vi "edit.vi"(8 "error in (no error)":errorcluster, 11 "TCSettings in":refnum<class "TCSettings.lvclass">) -> (0 "error out":errorcluster, 2 "cancelIsTrue out":bool, 3 "TCSettings out":refnum<class "TCSettings.lvclass">)   [LabVIEW 2016, in "Settings.lvlib" / "TCSettings.lvclass"]
uses:
  TCSettings.lvclass
  C:/Users/aanania/Documents/ts_monochromator_windows/MonoSettings/Settings/Settings/Setting.lvclass
  ConfigurationTypedefs/Base/MonochromatorSettings.ctl
  Typedefs/wavelength.ctl
  Typedefs/slitWidth.ctl
  ConfigurationTypedefs/Base/TCPConfiguration.ctl
  Settings/Setting.lvclass/Setting.ctl
  <vilib>/Utility/xml.llb/Write to XML File(string).vi
  Settings/Setting.lvclass
  ConfigurationTypedefs/ConfigurationTypedefs.lvlib
panel:
  in  "SettingTab":enum32{"TCP Settings", "Monochromator Limits"}(tab)
  in  "TCP Configuration":T1={"IP"="127.0.0.1", "port_low"=50000, "port_up"=50000, "connection_timeout "=10, "reading_timeout"=10, "writing_timeout"=10}
  in  "SetLimits":T2={"Force Init"=FALSE, "WavelengthMin"=300.0, "WavelengthMax"=800.0, "SlitWidthMin"=2.0, "SlitWidthMax"=7.0}
  out "String":string
  in  "cancelIsTrue":bool
  in  "saveIsTrue":bool
  in  "Listbox":i32(listbox)
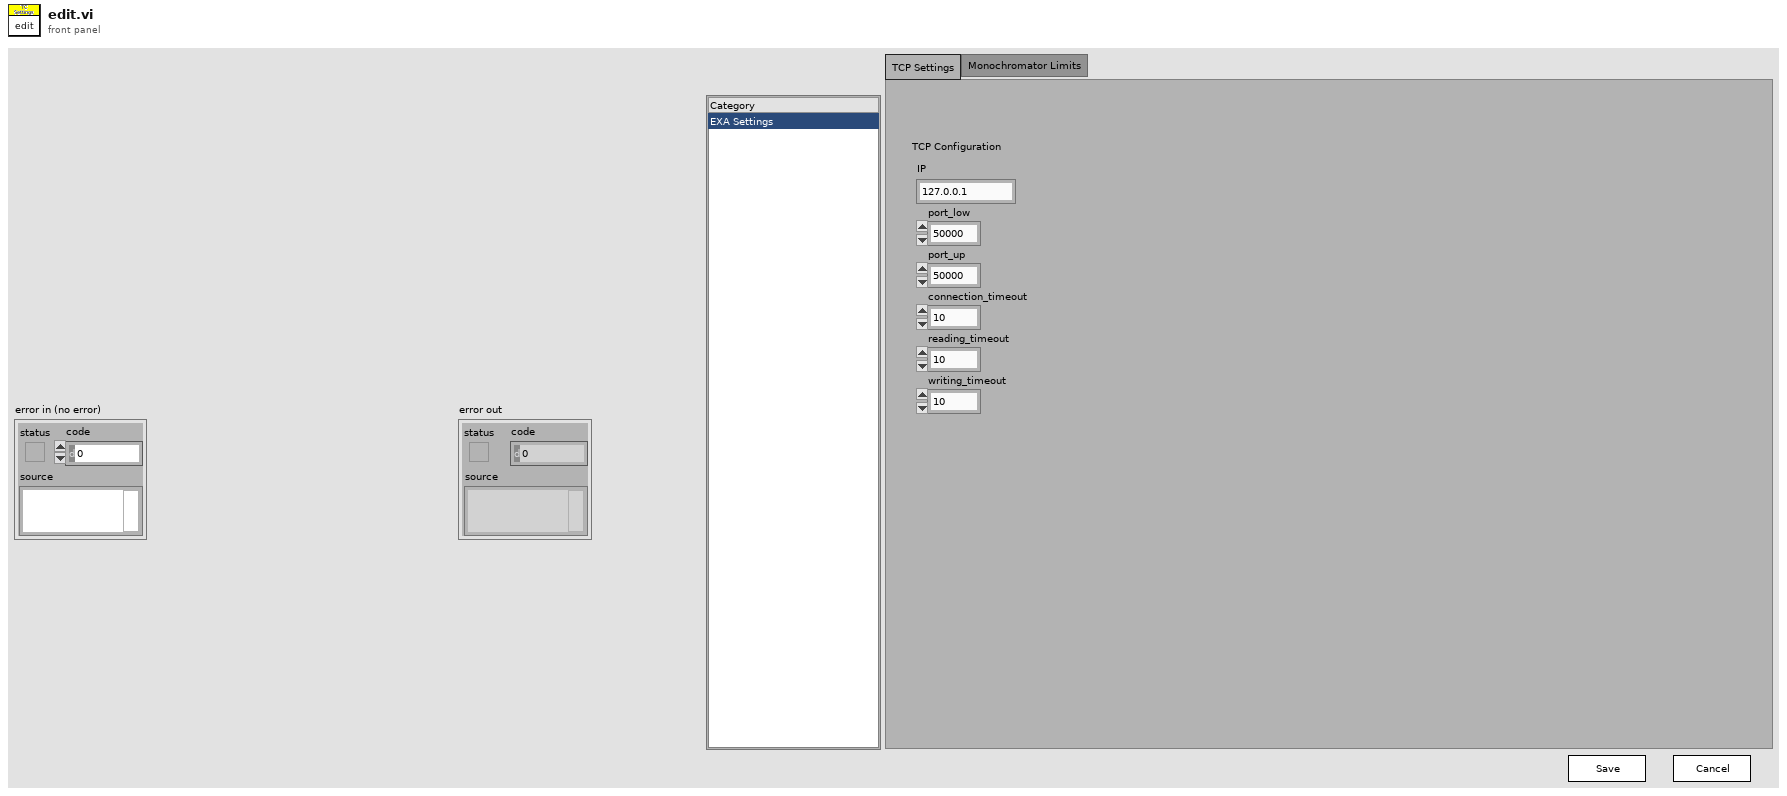
[diagram p1: front panel]
types:
  T1 = typedef "Settings.lvlib/ConfigurationTypedefs.lvlib/TCPConfiguration.ctl" = cluster{"IP":string, "port_low":u16, "port_up":u16, "connection_timeout ":i32, "reading_timeout":i32, "writing_timeout":i32}
  T2 = typedef "Settings.lvlib/ConfigurationTypedefs.lvlib/MonochromatorSettings.ctl" = cluster{"Force Init":bool, "WavelengthMin":T3, "WavelengthMax":T3, "SlitWidthMin":T4, "SlitWidthMax":T4}
  T3 = typedef "wavelength.ctl" = dbl
  T4 = typedef "slitWidth.ctl" = dbl
  T5 = enum32{"Invalid", "Standard", "Closed", "Hidden", "Minimized", "Maximized"}
  T6 = enum16{"open", "replace", "create", "open or create", "replace or create", "replace or create with confirmation"}
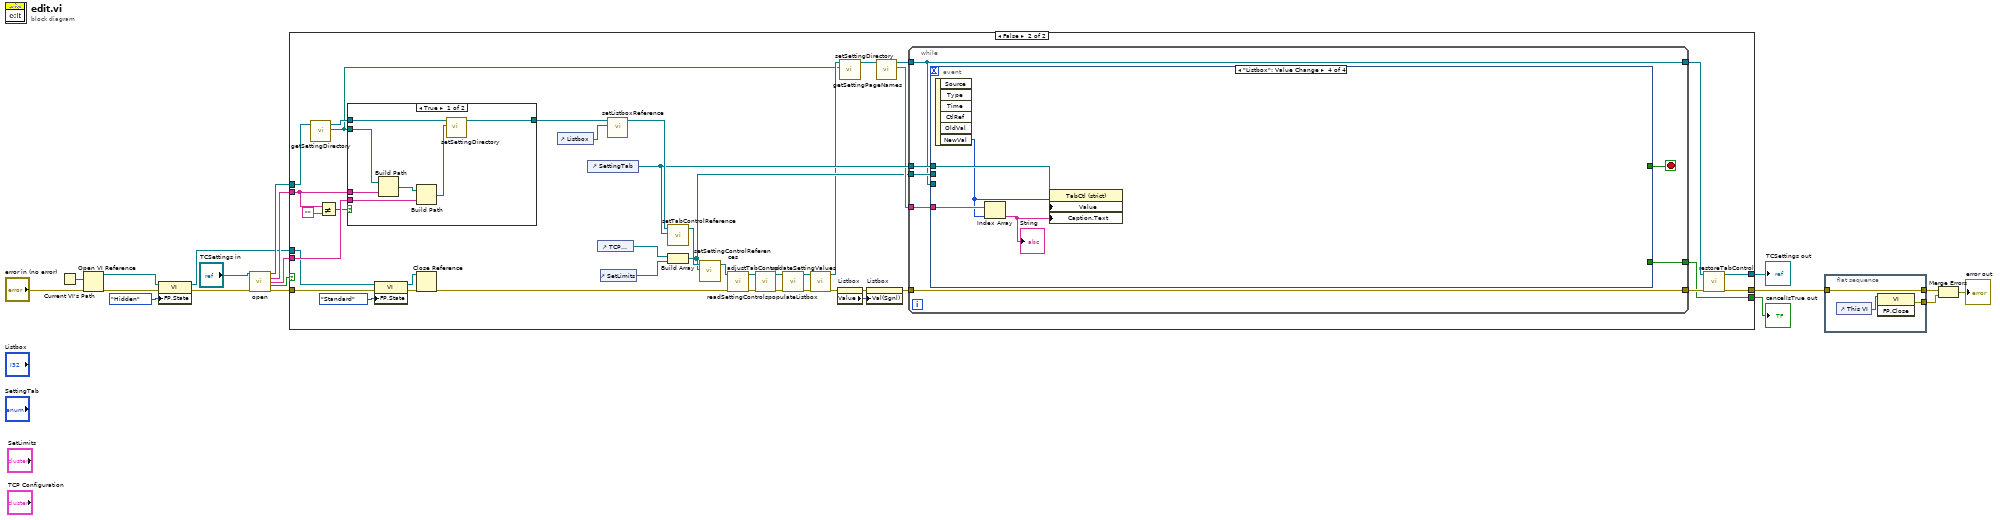
[diagram p0: block diagram]
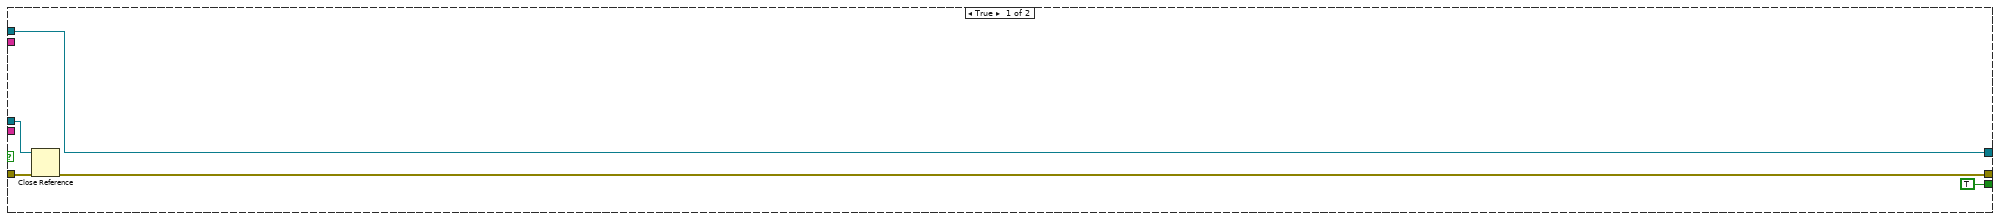
[diagram p2: hidden frame]
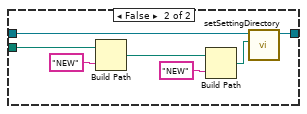
[diagram p3: hidden frame]
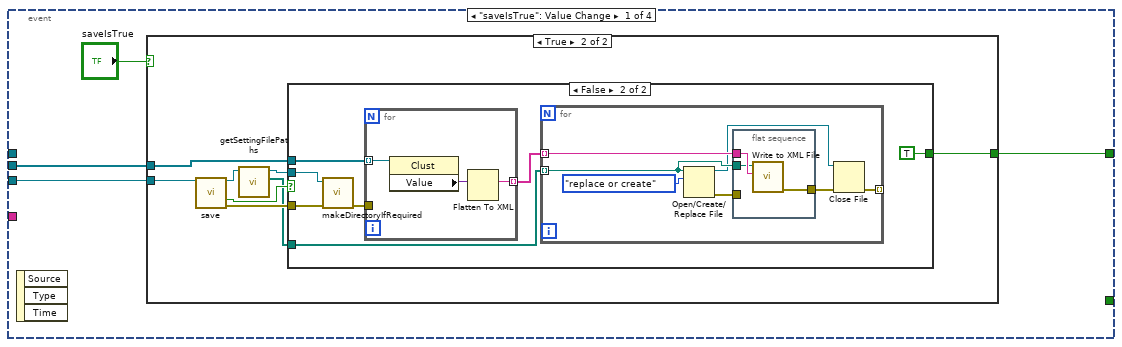
[diagram p4: hidden frame]
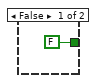
[diagram p5: hidden frame]
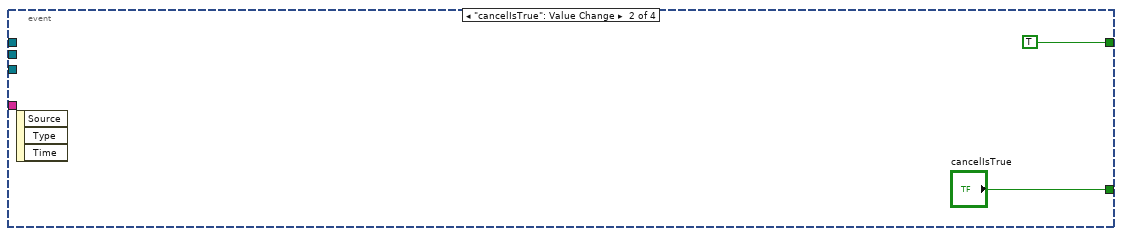
[diagram p7: hidden frame]
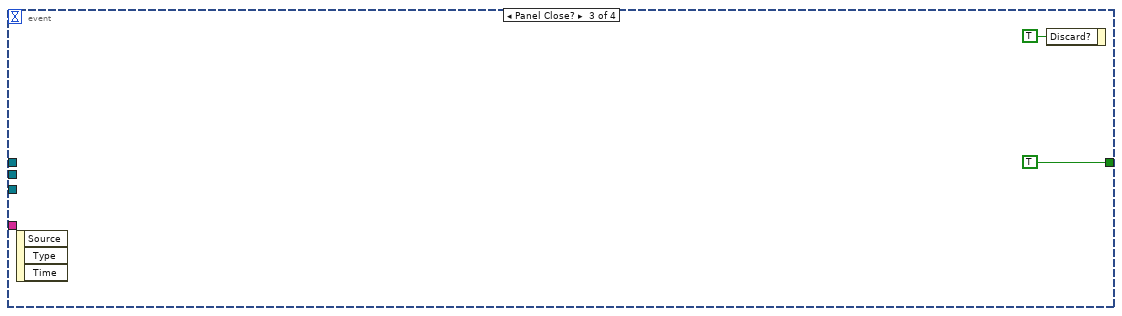
[diagram p8: hidden frame]
diagram:
  n1 = Current VI's Path() -> (path=w8:path)
  n2 = Open VI Reference(vi path=w8, error in (no error)="error in (no error)") -> (vi reference=w7:refnum<vi>, error out=w6:errorcluster)  [unwired: 4 in]
  n3 = property class="VI"(reference=w7, error in=w6, "FP.State"=T5."Hidden" ("Front Panel Window:State")) -> (reference out=w1:refnum<vi>, error out=w3:errorcluster)
  n4 = call "open.vi"("TCSettings in"="TCSettings in", "error in (no error)"=w3) -> ("TCSettings out"=w19:refnum<class "TCSettings.lvclass">, "SelectedSet"=w13:string, "SelectedVersion"=w15:string, "Canceled"=w11:bool, "error out"=w2:errorcluster)  [unwired: 9 in]
  n5 = case shown="False" w11 {
    tunnel: w19 -> [w24 w57]
    tunnel: w15 -> [_ w41]
    tunnel: [w24 w40] -> w9
    tunnel: [w20 w39] -> w14
    tunnel: w13 -> [_ w37]
    tunnel: [TRUE ("cancelIsTrue") w32] -> w12
    tunnel: w2 -> [w21 w26]
    tunnel: w1 -> [w22 w25]
    frame True {
      n6 = Close Reference(reference=w22, error in (no error)=w21) -> (error out=w20:errorcluster)
    }
    frame False {
      n7 = call "getSettingDirectory.vi"("BaseSetting in"=w57) -> ("SettingDirectory"=w33:path, "BaseSetting out"=w56:refnum<class "TCSettings.lvclass">)  [unwired: 9 in]
      n8 = Not Equal?(x=w37, y="") -> (x != y?=w36:bool)
      n9 = case shown="True" w36 {
        tunnel: w56 -> [w72 w79]
        tunnel: [w71 w78] -> w42
        tunnel: w41 -> [w69 _]
        tunnel: w33 -> [w67 w75]
        tunnel: w37 -> [w66 _]
        frame True {
          n10 = Build Path(base path=w67, name or relative path=w66) -> (appended path=w70:path)
          n11 = Build Path(base path=w70, name or relative path=w69) -> (appended path=w68:path)
          n12 = call "setSettingDirectory.vi"("SettingDirectory"=w68, "BaseSetting in"=w72) -> ("BaseSetting out"=w71:refnum<class "TCSettings.lvclass">)  [unwired: 9 in]
        }
        frame False {
          n13 = Build Path(base path=w75, name or relative path="NEW") -> (appended path=w77:path)
          n14 = Build Path(base path=w77, name or relative path="NEW") -> (appended path=w76:path)
          n15 = call "setSettingDirectory.vi"("SettingDirectory"=w76, "BaseSetting in"=w79) -> ("BaseSetting out"=w78:refnum<class "TCSettings.lvclass">)  [unwired: 9 in]
        }
      }
      n16 = property class="VI"(reference=w25, error in=w26, "FP.State"=T5."Standard" ("Front Panel Window:State")) -> (reference out=w29:refnum<vi>, error out=w30:errorcluster)
      n17 = Close Reference(reference=w29, error in (no error)=w30) -> (error out=w27:errorcluster)
      n18 = control-ref of="Listbox"() -> (w59:refnum<vi>)
      n19 = control-ref of="SettingTab"() -> (w49:refnum<vi>)
      n20 = control-ref of="TCP Configuration"() -> (w58:refnum<vi>)
      n21 = control-ref of="SetLimits"() -> (w31:refnum<vi>)
      n22 = call "setListboxReference.vi"("ListboxReference"=w59, "Setting in"=w42) -> ("Setting out"=w60:refnum<class "TCSettings.lvclass">)  [unwired: 9 in]
      n23 = call "setTabControlReference.vi"("TabControlReference"=w49, "Setting in"=w60) -> ("Setting out"=w61:refnum<class "TCSettings.lvclass">)  [unwired: 9 in]
      n24 = Build Array(w58, w31) -> (w46:refnum<vi>[])
      n25 = call "setSettingControlReferences.vi"("SettingControlReferences"=w46, "Setting in"=w61) -> ("Setting out"=w62:refnum<class "TCSettings.lvclass">)  [unwired: 9 in]
      n26 = call "readSettingControls.vi"("error in (no error)"=w27, "BaseSetting in"=w62) -> ("error out"=w52:errorcluster, "BaseSetting out"=w63:refnum<class "TCSettings.lvclass">)  [unwired: 8 in]
      n27 = call "adjustTabControl.vi"("error in (no error)"=w52, "BaseSetting in"=w63) -> ("error out"=w51:errorcluster, "BaseSetting out"=w64:refnum<class "TCSettings.lvclass">)  [unwired: 8 in]
      n28 = call "populateListbox.vi"("error in (no error)"=w51, "BaseSetting in"=w64) -> ("error out"=w50:errorcluster, "BaseSetting out"=w65:refnum<class "TCSettings.lvclass">)  [unwired: 8 in]
      n29 = call "updateSettingValues.vi"("error in (no error)"=w50, "BaseSetting in"=w65) -> ("error out"=w53:errorcluster, "BaseSetting out"=w35:refnum<class "TCSettings.lvclass">)  [unwired: 8 in]
      n30 = property on="Listbox" class="LstBox (strict)"(error in=w53) -> (error out=w55:errorcluster, "Value"=w54:i32)  [unwired: 1 in, 1 out]
      n31 = call "setSettingDirectory.vi"("SettingDirectory"=w33, "BaseSetting in"=w35) -> ("BaseSetting out"=w34:refnum<class "TCSettings.lvclass">)  [unwired: 9 in]
      n32 = property on="Listbox" class="LstBox (strict)"(error in=w55, "Val(Sgnl)"=w54) -> (error out=w45:errorcluster)  [unwired: 1 in, 1 out]
      n33 = call "getSettingPageNames.vi"("Setting in"=w34) -> ("SettingPageNames"=w47:string[], "Setting out"=w48:refnum<class "TCSettings.lvclass">)  [unwired: 9 in]
      n34 = while {
        tunnel: w49 -> [w84]
        tunnel: w46 -> [w86]
        tunnel: [w81] -> w43
        tunnel: w48 -> [w81]
        tunnel: w45 -> [w83]
        tunnel: [w83] -> w44
        tunnel: [w82] -> w32
        tunnel: w47 -> [w80]
        stop <- w85 stop-if-true
        n35 = event shown="[3] \"Listbox\": Value Change" {
          selector: _ -> [_ _ _ _]
          dyn-events: _ -> [_ _ _ _]
          timeout: _ -> [_ _ _ _]
          tunnel: [w88 TRUE TRUE _] -> w85
          tunnel: w80 -> [_ _ _ w126]
          tunnel: w84 -> [_ _ _ w127]
          tunnel: w86 -> [w90 _ _ _]
          tunnel: [_ "cancelIsTrue" _ _] -> w82
          tunnel: w81 -> [w89 _ _ _]
          event "saveIsTrue": Value Change {
            n36 = event-data() -> ()  [unwired: 1 in, 3 out]
            n37 = case shown="True" "saveIsTrue" {
              tunnel: w90 -> [_ w99]
              tunnel: w89 -> [_ w98]
              tunnel: [FALSE w96] -> w88
              frame False {
              }
              frame True {
                n38 = call "save.vi"("M1M3Settings in"=w98) -> ("M1M3Settings out"=w94:refnum<class "TCSettings.lvclass">, "Canceled"=w95:bool, "error out"=w97:errorcluster)  [unwired: 12 in]
                n39 = call "getSettingFilePaths.vi"("Setting in"=w94) -> ("SettingFilePaths"=w92:path[], "Setting out"=w93:refnum<class "TCSettings.lvclass">)  [unwired: 9 in]
                n40 = case shown="False" w95 {
                  tunnel: w92 -> [_ w106]
                  tunnel: w99 -> [_ w105]
                  tunnel: w93 -> [_ w102]
                  tunnel: w97 -> [_ w101]
                  tunnel: [_ TRUE] -> w96
                  frame True {
                  }
                  frame False {
                    n41 = call "makeDirectoryIfRequired.vi"("error in (no error)"=w101, "BaseSetting in"=w102) -> ("error out"=w103:errorcluster)  [unwired: 8 in, 1 out]
                    n42 = for {
                      tunnel: w105 -> [w119] mode=indexing
                      tunnel: [w117] -> w104 mode=indexing
                      tunnel: w103 -> [_]
                      n43 = property class="Clust"(reference=w119) -> ("Value"=w118:variant)  [unwired: 1 in, 2 out]
                      n44 = Flatten To XML(anything=w118) -> (xml string=w117:string)
                    }
                    n45 = for {
                      tunnel: w106 -> [w110] mode=indexing
                      tunnel: w104 -> [w113] mode=indexing
                      tunnel: [w107] -> _ mode=indexing
                      n46 = Open/Create/Replace File(file path (use dialog)=w110, operation (0:open)=T6."replace or create") -> (refnum out=w109:refnum<file>, error out=w111:errorcluster)  [unwired: 4 in, 1 out]
                      n47 = flat-sequence {
                        tunnel: w113 -> [w116]
                        tunnel: [w115] -> w108
                        tunnel: w111 -> [_]
                        tunnel: w110 -> [w114]
                        frame #0 {
                          n48 = call-poly <vilib>:"Write to XML File.vi"("XML Input"=w116, "XML File Path"=w114) -> ("error out"=w115:errorcluster)  [unwired: 7 in, 2 out]
                        }
                      }
                      n49 = Close File(refnum=w109, error in=w108) -> (error out=w107:errorcluster)  [unwired: 1 out]
                    }
                  }
                }
              }
            }
          }
          event "cancelIsTrue": Value Change {
            n50 = event-data() -> ()  [unwired: 1 in, 3 out]
          }
          event Panel Close? {
            n51 = event-data() -> ()  [unwired: 1 in, 3 out]
            n52 = event-data("Discard?"=TRUE) -> ()  [unwired: 1 in, 1 out]
          }
          event "Listbox": Value Change {
            n53 = event-data() -> ("NewVal"=w125:i32)  [unwired: 1 in, 5 out]
            n54 = Index Array(array=w126, index=w125) -> (element=w124:string)
            "String" <- w124
            n55 = property class="TabCtl (strict)"(reference=w127, "Value"=w125, "Caption.Text"=w124) -> ()  [unwired: 1 in, 2 out]
          }
        }
      }
      n56 = call "restoreTabControl.vi"("error in (no error)"=w44, "BaseSetting in"=w43) -> ("error out"=w39:errorcluster, "BaseSetting out"=w40:refnum<class "TCSettings.lvclass">)  [unwired: 8 in]
    }
  }
  "cancelIsTrue out" <- w12
  "TCSettings out" <- w9
  n57 = flat-sequence {
    tunnel: [w129] -> w18
    tunnel: [w128] -> w17
    tunnel: w14 -> [w128]
    frame #0 {
      n58 = control-ref of="This VI"() -> (w130:refnum<vi>)
      n59 = invoke class="VI" method="FP.Close"(reference=w130) -> (error out=w129:errorcluster)  [unwired: 2 in, 2 out]
    }
  }
  n60 = Merge Errors(w17, w18) -> (→"error out":errorcluster)
